vi "Update Nimbelink database field.vi"(6 "New data string":string, 7 "Part Number":string, 8 "error in (no error)":errorcluster, 9 "Dbase field to change":T1 items=["work_order", "btw_sn", "mac", "meid", "operator", "date_time", "part_number", "imei", "sim_id", "phone_number", "test_result", "board_sn", "test_time", "test_program", "test_version", "sent_data_to_customer", "device_type", "guid", "firmware_rev", "msn", "extra5", "test_pc_name", "extra7", "extra8", "extra9", "extra10", "extra11", "extra12", "PN Rev"], 10 "Lookup field data":string, 11 "Dbase field to lookup by":T1 items=["work_order", "btw_sn", "mac", "meid", "operator", "date_time", "part_number", "imei", "sim_id", "phone_number", "test_result", "board_sn", "test_time", "test_program", "test_version", "sent_data_to_customer", "device_type", "guid", "firmware_rev", "msn", "extra5", "test_pc_name", "extra7", "extra8", "extra9", "extra10", "extra11", "extra12", "PN Rev"]) -> (0 "error out":errorcluster)   [LabVIEW 2013]
uses:
  Nimbelink database fields.ctl
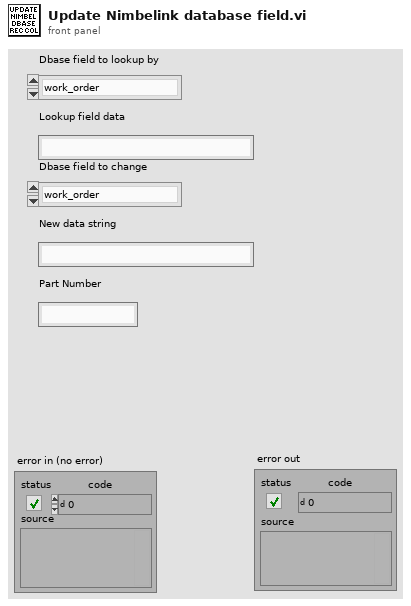
[diagram p1: front panel]
types:
  T1 = typedef "Nimbelink database fields.ctl" = u16
  T2 = enum16{"Query", "Insert", "Select", "Dump Recs", "Get Rec Count", "Get Col Names", "Insert all fields", "Find", "Get last test result"}
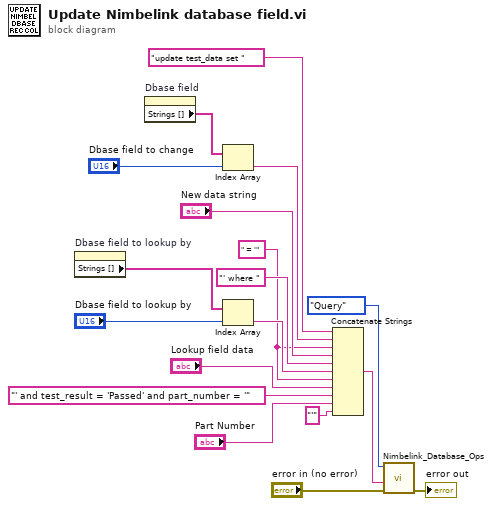
[diagram p0: block diagram]
diagram:
  w6 = " = '" ("string")
  n1 = property on="Dbase field to lookup by" class="Ring (strict)"() -> ("Strings []"=w9:string[])  [unwired: 2 in, 2 out]
  n2 = property on="Dbase field" class="Ring (strict)"() -> ("Strings []"=w17:string[])  [unwired: 2 in, 2 out]
  n3 = Index Array(array=w17, index="Dbase field to change") -> (element=w14:string)
  n4 = Index Array(array=w9, index="Dbase field to lookup by") -> (element=w7:string)
  n5 = Concatenate Strings("update test_data set " ("string"), w14, w6, "New data string", "' where " ("string"), w7, w6, "Lookup field data", "' and test_result = 'Passed' and part_number = '" ("string"), "Part Number", "'" ("string")) -> (w4:string)
  n6 = call "Nimbelink_Database_Ops.vi"("Error in (no error)"="error in (no error)", "SQL Query"=w4, "Operation"=T2."Query") -> ("Error out"=→"error out":errorcluster)  [unwired: 3 in, 5 out]
